vi "svl_Running Equivalent Continuous Resampled Level (N Ch).vi"(6 "integration time [s]":dbl format="%.2f", 8 "error in (no error)":errorcluster, 9 "processing state":T2(ring), 11 "scaled signals [EU]":T1(array[cluster])=[{"r0"=0.0, "dr"=0.0, "even angle signal"=[]}] {"even angle signal" format="%.2f"; "dr" format="%.2f"; "r0" format="%.2f"}) -> (0 "error out":errorcluster, 3 "energy level [ ] [EU^2 rms]":dbl[](array[numeric]) format="%.2f", 4 "actual integration time [s]":dbl=125.0 format="%.2f")   [LabVIEW 2017]
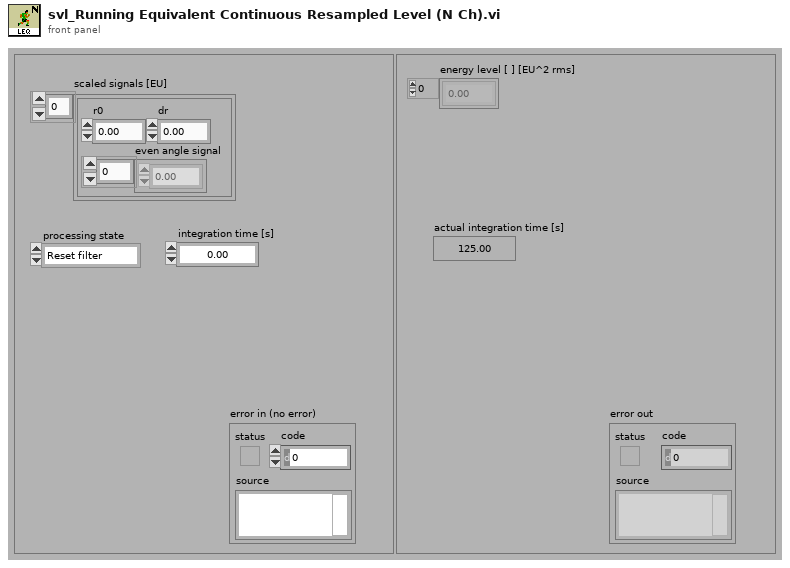
[diagram p1: front panel]
types:
  T1 = cluster{"r0":dbl, "dr":dbl, "even angle signal":dbl[]}[]
  T2 = enum16{"Reset filter", "Restart averaging", "Continue processing"}
  T3 = cluster{"r0":dbl, "dr":dbl, "even angle signal":dbl[]}
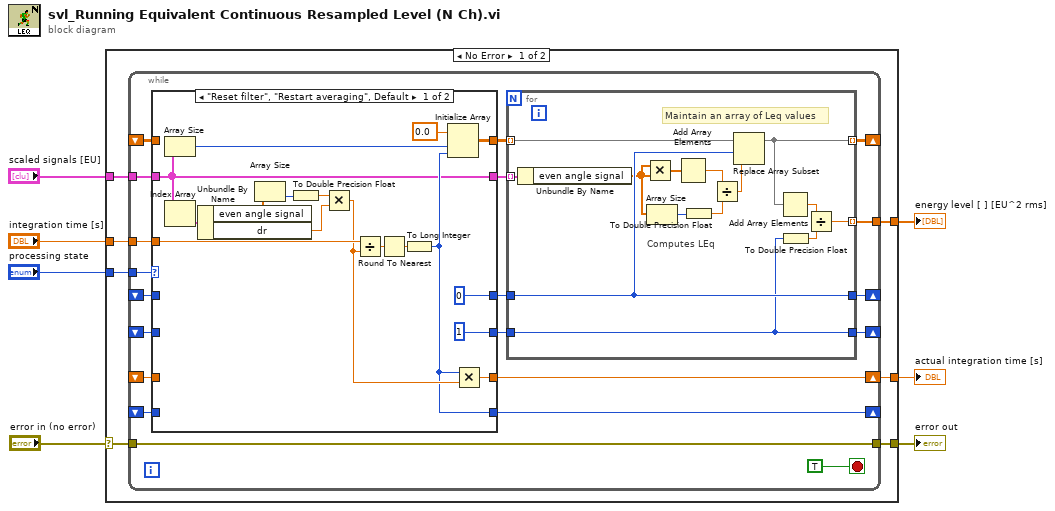
[diagram p0: block diagram]
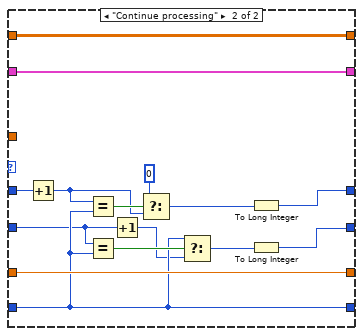
[diagram p2: hidden frame]
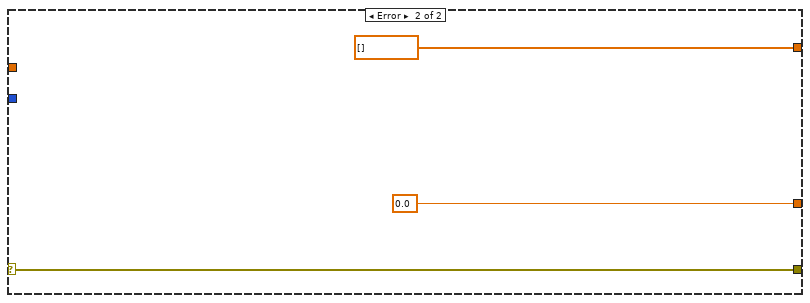
[diagram p3: hidden frame]
diagram:
  n1 = case shown="No Error" "error in (no error)" {
    selector: "error in (no error)" -> [w8 w83]
    tunnel: "integration time [s]" -> [w14 _]
    tunnel: "scaled signals [EU]" -> [w13 _]
    tunnel: "processing state" -> [w12 _]
    tunnel: [w11 dbl[] []] -> w3
    tunnel: [w10 0.0] -> w2
    tunnel: [w9 w83] -> w1
    frame No Error {
      n2 = while {
        shift-left: _ -> [w15]
        shift-right: [w16] -> _
        tunnel: w8 -> [w17]
        tunnel: [w17] -> w9
        shift-left: _ -> [w18]
        shift-right: [w19] -> w10
        shift-left: _ -> [w20]
        shift-right: [w21] -> _
        shift-left: _ -> [w23]
        shift-right: [w24] -> _
        tunnel: [w26] -> w11
        shift-left: _ -> [w27]
        shift-right: [w28] -> _
        tunnel: w14 -> [w31]
        tunnel: w12 -> [w33]
        tunnel: w13 -> [w32]
        stop <- TRUE stop-if-true
        n3 = case shown="\"Reset filter\", \"Restart averaging\", Default" w33 {
          tunnel: w32 -> [w39 w66]
          tunnel: w31 -> [w43 _]
          tunnel: [w39 w66] -> w30
          tunnel: [w51 w65] -> w29
          tunnel: w27 -> [_ w65]
          tunnel: [0 ("t") w58] -> w25
          tunnel: w23 -> [_ w62]
          tunnel: [1 ("t") w55] -> w22
          tunnel: w20 -> [_ w53]
          tunnel: [w44 w61] -> w19
          tunnel: w18 -> [_ w61]
          tunnel: [w41 w54] -> w16
          tunnel: w15 -> [_ w54]
          frame "Reset filter", "Restart averaging", Default {
            n4 = Array Size(array=w39) -> (size(s)=w40:i32)
            n5 = Index Array(array=w39) -> (element=w37:T3)  [unwired: 1 in]
            n6 = Unbundle By Name(w37) -> ("even angle signal"=w35:dbl[], "dr"=w36:dbl)
            n7 = Array Size(array=w35) -> (size(s)=w38:i32)
            n8 = To Double Precision Float(number=w38) -> (double precision float=w48:dbl)
            n9 = Multiply(x=w48, y=w36) -> (x*y=w42:dbl)
            n10 = Divide(x=w43, y=w42) -> (x/y=w47:dbl)
            n11 = Round To Nearest(number=w47) -> (nearest integer value=w46:dbl)
            n12 = To Long Integer(number=w46) -> (32bit integer=w41:i32)
            n13 = Initialize Array(0.0 ("duration (sec)"), w40, w41) -> (w51:dbl[][])
            n14 = Multiply(x=w41, y=w42) -> (x*y=w44:dbl)
          }
          frame "Continue processing" {
            n15 = Increment(x=w62) -> (x+1=w59:i32)
            n16 = Equal?(x=w59, y=w54) -> (x = y?=w60:bool)
            n17 = Equal?(x=w53, y=w54) -> (x = y?=w57:bool)
            n18 = Increment(x=w53) -> (x+1=w52:i32)
            n19 = Select(t=0, s=w60, f=w59) -> (s? t:f=w63:i32)
            n20 = Select(t=w54, s=w57, f=w52) -> (s? t:f=w56:i32)
            n21 = To Long Integer(number=w63) -> (32bit integer=w58:i32)
            n22 = To Long Integer(number=w56) -> (32bit integer=w55:i32)
          }
        }
        n23 = for {
          tunnel: w30 -> [w68] mode=indexing
          tunnel: w29 -> [w73] mode=indexing
          tunnel: [w72] -> w28 mode=indexing
          tunnel: [w71] -> w26 mode=indexing
          tunnel: w25 -> [w70]
          tunnel: [w70] -> w24
          tunnel: w22 -> [w69]
          tunnel: [w69] -> w21
          # "Maintain an array of Leq values"
          # "Computes LEq"
          n24 = Unbundle By Name(w68) -> ("even angle signal"=w67:dbl[])
          n25 = Multiply(x=w67, y=w67) -> (x*y=w75:dbl[])
          n26 = Array Size(array=w67) -> (size(s)=w79:i32)
          n27 = Add Array Elements(numeric array=w75) -> (sum=w80:dbl)
          n28 = To Double Precision Float(number=w79) -> (double precision float=w78:dbl)
          n29 = Divide(x=w80, y=w78) -> (x/y=w74:dbl)
          n30 = Replace Array Subset(array=w73, new element=w74, index=w70) -> (w72:dbl[])
          n31 = Add Array Elements(numeric array=w72) -> (sum=w77:dbl)
          n32 = To Double Precision Float(number=w69) -> (double precision float=w76:dbl)
          n33 = Divide(x=w77, y=w76) -> (x/y=w71:dbl)
        }
      }
    }
    frame Error {
    }
  }
  "error out" <- w1
  "energy level [ ] [EU^2 rms]" <- w3
  "actual integration time [s]" <- w2
